vi "json step editor proto.vi"() -> ()   [LabVIEW 2020]
uses:
  controls/PROTO_stepV2.ctl
  controls/step_type.ctl
  controls/write_read.ctl
panel:
  in  "save":bool
  out "steps array out":T1[](array[typedef]) {"data num" format="%.3f"}
  in  "exit without saving":bool
  in  "steps array out":T1[](array[typedef]) {"data num" format="%.3f"}
  in  "exit and save":bool
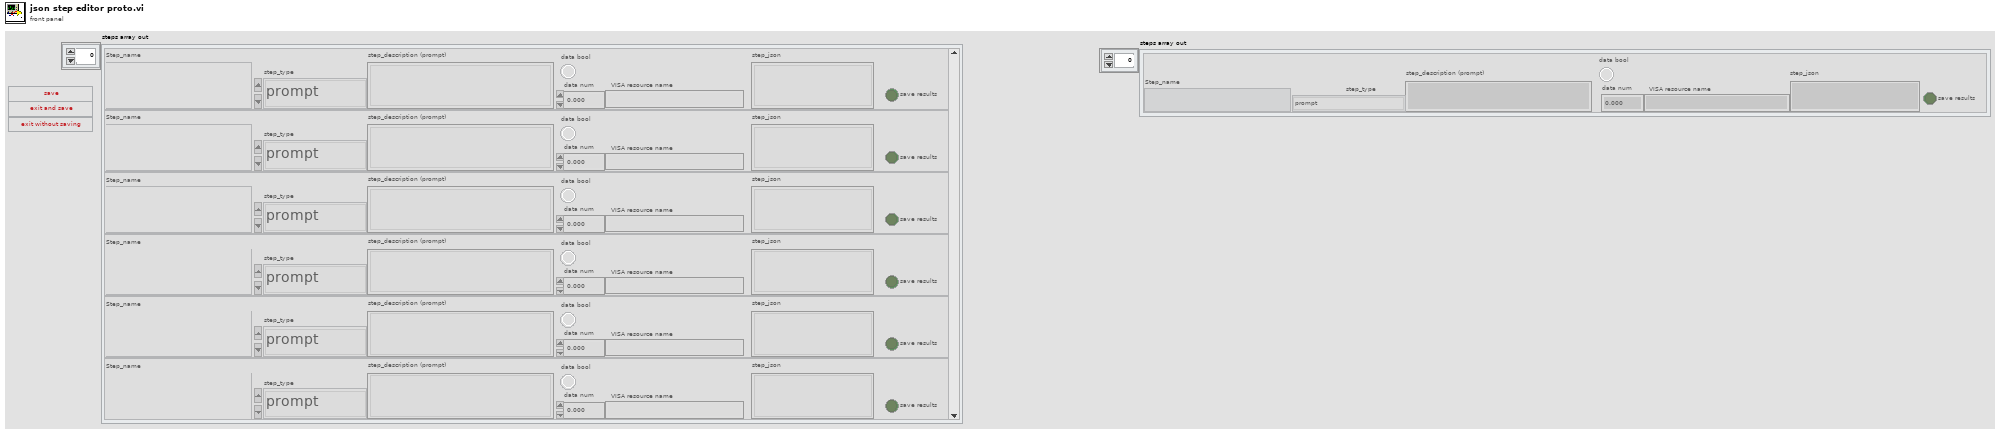
[diagram p1: front panel]
types:
  T1 = typedef "PROTO_stepV2.ctl" = cluster{"VISA resource name":string, "data num":dbl, "step_description (prompt)":string, "step_json":string, "save results":bool, "step_type":T2, "Step_name":string, "data bool":bool}
  T2 = typedef "step_type.ctl" = enum16{"default", "prompt", "sequence#", "12V_1_power supply on_off", "12V_2_power supply on_off", "set_hipot_V", "set_hipot_I_limit", "set_hipot_ramping (sec)", "set hipot_hold_time", "read_hipot_V", "read_hipot_I", "set_daq", "read_daq", "flash uds", "wait (sec)", "record_pass_fail", "ac_charge_test", "dc_400V_charging", "HAPS Heater Output", "HAPS Compressor Output", "stop_test", "error_exit"}
  T3 = typedef "write_read.ctl" = enum16{"write", "read"}
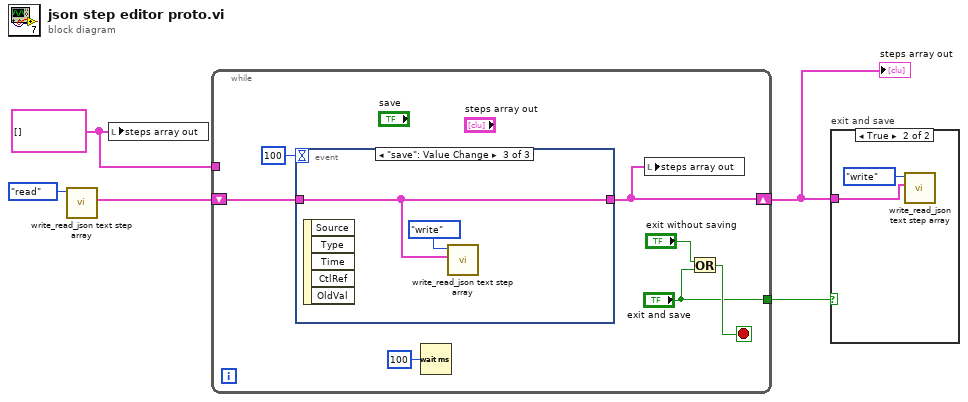
[diagram p0: block diagram]
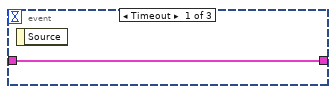
[diagram p3: hidden frame]
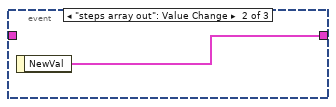
[diagram p4: hidden frame]
diagram:
  w2 = T1[] [] ("steps array out")
  n1 = call "write_read_json text step array.vi"("write_read"=write_read."read") -> ("steps array out"=w4:T1[])  [unwired: 9 in, 1 out]
  n2 = local write "steps array out"(w2) -> ()
  n3 = while {
    shift-right: [w9] -> w1
    shift-left: w4 -> [w11]
    tunnel: ["exit and save"] -> w3
    tunnel: w2 -> [_]
    stop <- w8 stop-if-true
    n4 = event shown="[2] \"save\": Value Change" {
      selector: _ -> [_ _ _]
      dyn-events: _ -> [_ _ _]
      timeout: 100 -> [_ _ _]
      tunnel: w11 -> [w13 _ w15]
      tunnel: [w13 w14 w15] -> w9
      event Timeout {
        n5 = event-data() -> ()  [unwired: 1 in, 1 out]
      }
      event "steps array out": Value Change {
        n6 = event-data() -> ("NewVal"=w14:T1[])  [unwired: 1 in]
      }
      event "save": Value Change {
        n7 = event-data() -> ()  [unwired: 1 in, 5 out]
        n8 = call "write_read_json text step array.vi"("json_array_from_file"=w15, "write_read"=write_read."write") -> ()  [unwired: 8 in, 2 out]
      }
    }
    n9 = Wait (ms)(milliseconds to wait=u32 100) -> ()  [unwired: 1 out]
    n10 = local write "steps array out"(w9) -> ()
    n11 = Or(x="exit without saving", y="exit and save") -> (x .or. y?=w8:bool)
  }
  "steps array out" <- w1
  n12 = case "exit and save" shown="True" w3 {
    tunnel: w1 -> [_ w17]
    frame False {
    }
    frame True {
      n13 = call "write_read_json text step array.vi"("json_array_from_file"=w17, "write_read"=write_read."write") -> ()  [unwired: 8 in, 2 out]
    }
  }
